vi "Digital PWM In Settings.vi"() -> ()   [LabVIEW 2019]
uses:
  Submodules/Source/Types/PWM.Measure.Digital.Settings.ctl
  <vilib>/rvi/Emulation/niFpgaGetClockAttributes.vi
  <vilib>/rvi/Emulation/niFpgaSctlEmulationGetInTimedLoop.vi
  <vilib>/rvi/Emulation/niFpgaEmulationReportErrorSimple.vi
  <vilib>/rvi/Emulation/niFpgaCriticalErrorInLSC.vi
  Submodules/Source/Speciality FPGA IO.lvlib
panel:
  out "TIMEOUT":u32
  out "ACTIVE EDGE":bool
  in  "Digital PWM In Settings":T1
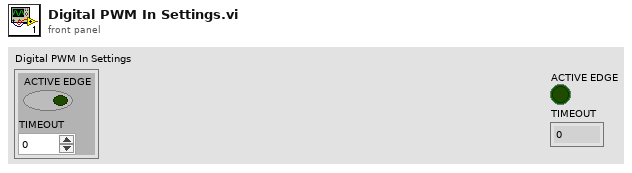
[diagram p1: front panel]
types:
  T1 = typedef "Speciality FPGA IO.lvlib/PWM.Measure.Digital.Settings.ctl" = cluster{"ACTIVE EDGE":bool, "TIMEOUT":u32}
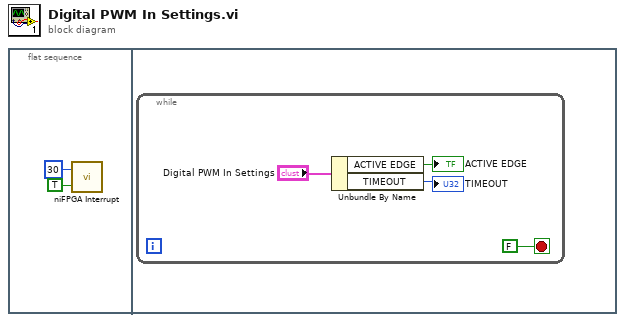
[diagram p0: block diagram]
diagram:
  n1 = flat-sequence {
    frame #0 {
      n2 = call <vilib>:"niFPGA Interrupt.vi"("Wait Until Cleared (F)"=TRUE, "IRQ Number (0)"=u8 30) -> ()  [unwired: 1 in]
    }
    frame #1 {
      n3 = while {
        stop <- FALSE stop-if-true
        n4 = Unbundle By Name("Digital PWM In Settings") -> ("ACTIVE EDGE"=→"ACTIVE EDGE":bool, "TIMEOUT"=→"TIMEOUT":u32)
      }
    }
  }
